vi "test.vi"() -> ()   [LabVIEW 2017]
uses:
  <vilib>/myRIO/Common/Instrument Driver Framework/myRIO v1.0/Encoder/typedefs/Encoder Signal Mode.ctl
  <vilib>/myRIO/Instrument Drivers/Onboard IO/PWM/typedefs/PWM Reference.ctl
  <vilib>/myRIO/Common/Instrument Driver Framework/Utilities/typedefs/myRIO Generic Hardware Reference.ctl
  <vilib>/myRIO/Common/Instrument Driver Framework/Utilities/typedefs/Hardware Version Enum.ctl
  <vilib>/myRIO/Common/Instrument Driver Framework/Utilities/typedefs/myRIO v1.0 Reference.ctl
  <vilib>/myRIO/Common/Instrument Driver Framework/Utilities/typedefs/Generic FPGA Reference.ctl
  <vilib>/myRIO/Common/Instrument Driver Framework/myRIO v1.0/PWM/typedefs/PWM Channels Enum.ctl
  <vilib>/myRIO/Instrument Drivers/Onboard IO/PWM/typedefs/PWM Configuration.ctl
  <vilib>/userdefined/High Color/nirio_resource_hc.ctl
  <vilib>/myRIO/Instrument Drivers/Onboard IO/DIO/typedefs/DIO Reference.ctl
  <vilib>/myRIO/Common/Instrument Driver Framework/myRIO v1.0/DIO/typedefs/DIO Channels List.ctl
  <vilib>/myRIO/Common/Instrument Driver Framework/myRIO v1.0/DIO/typedefs/DIO Channels Enum.ctl
  <vilib>/myRIO/Common/Instrument Driver Framework/Utilities/vis/Is FPGA Ref Available.vi
  <vilib>/myRIO/Common/Instrument Driver Framework/myRIO v1.0/PWM/vis/myRIO v1.1 Open PWM.vi
  <vilib>/myRIO/Instrument Drivers/Onboard IO/PWM/vis/Set Duty Cycle and Frequency.vi
  <vilib>/myRIO/Common/Instrument Driver Framework/myRIO v1.0/DIO/vis/myRIO v1.1 Open DIO.vi
  <vilib>/myRIO/Instrument Drivers/Onboard IO/DIO/vis/Write.vi
  <vilib>/myRIO/Common/Instrument Driver Framework/Utilities/vis/Validate Channels.vi
  <vilib>/myRIO/Common/Instrument Driver Framework/myRIO v1.0/PWM/vis/myRIO v1.0 Reserve PWM.vi
  <vilib>/myRIO/Common/Instrument Driver Framework/myRIO v1.0/DIO/vis/myRIO v1.0 Reserve DIO.vi
  <vilib>/myRIO/Common/Instrument Driver Framework/myRIO v1.0/Encoder/vis/myRIO v1.0 Close Encoder.vi
  <vilib>/myRIO/Common/Instrument Driver Framework/myRIO v1.0/UART/vis/myRIO v1.0 Close UART.vi
  <vilib>/myRIO/Common/Instrument Driver Framework/myRIO v1.0/PWM/vis/myRIO v1.0 Build MUX Configuration PWM.vi
  <vilib>/myRIO/Common/Instrument Driver Framework/myRIO v1.0/Resource Manager/vis/myRIO v1.0 Reserve Channel List.vi
  <vilib>/myRIO/Common/Instrument Driver Framework/myRIO v1.0/DIO/vis/myRIO v1.0 Build MUX Configuration DIO.vi
  <vilib>/myRIO/Common/Instrument Driver Framework/myRIO v1.0/Encoder/vis/myRIO v1.0 Unreserve Encoder.vi
  <vilib>/myRIO/Common/Instrument Driver Framework/myRIO v1.0/Resource Manager/vis/myRIO v1.0 Create Configuration List.vi
  <vilib>/myRIO/Common/Instrument Driver Framework/myRIO v1.0/Resource Manager/vis/myRIO v1.0 Reserve Channel.vi
  <vilib>/myRIO/Common/Instrument Driver Framework/myRIO v1.0/Resource Manager/vis/myRIO v1.0 Unreserve Channel.vi
  <vilib>/myRIO/Common/Instrument Driver Framework/myRIO v1.0/Encoder/vis/myRIO v1.0 Build MUX Configuration Encoder.vi
  <vilib>/myRIO/Common/Instrument Driver Framework/myRIO v1.0/Resource Manager/vis/myRIO v1.0 Unreserve Channel List.vi
  <vilib>/myRIO/Common/Instrument Driver Framework/myRIO v1.0/Resource Manager/vis/myRIO v1.0 Build Mutex Name.vi
  <vilib>/Utility/error.llb/Error Cluster From Error Code.vi
  <vilib>/myRIO/Common/Instrument Driver Framework/myRIO v1.0/Encoder/vis/myRIO v1.0 Reset Encoder.vi
  <vilib>/Utility/VariantDataType/GetNumericInfo.vi
  <vilib>/myRIO/Common/Instrument Driver Framework/myRIO v1.0/myRIO v1.1 Open.vi
  <vilib>/myRIO/Common/Instrument Driver Framework/Utilities/vis/IO Manager.vi
  <vilib>/myRIO/Common/Instrument Driver Framework/Utilities/vis/Configuration Manager.vi
  <vilib>/myRIO/Common/Instrument Driver Framework/myRIO v1.0/Resource Manager/vis/myRIO v1.0 Configure IO.vi
  <vilib>/myRIO/Common/Instrument Driver Framework/myRIO v1.0/myRIO v1.0 Close.vi
  <vilib>/myRIO/Common/Instrument Driver Framework/myRIO v1.0/PWM/vis/myRIO v1.0 Write PWM.vi
  <vilib>/myRIO/Common/Instrument Driver Framework/myRIO v1.0/DIO/vis/myRIO v1.0 Write DIO.vi
  <vilib>/myRIO/Common/Instrument Driver Framework/myRIO v1.0/Encoder/vis/myRIO v1.0 Read Encoder.vi
  <vilib>/myRIO/Common/Instrument Driver Framework/myRIO v1.0/Encoder/vis/myRIO v1.0 Shutdown Encoder.vi
  <vilib>/myRIO/Common/Instrument Driver Framework/Utilities/vis/FPGA Ref Manager.vi
  <vilib>/myRIO/Common/Instrument Driver Framework/myRIO v1.0/myRIO v1.0 Reset FPGA.vi
  <vilib>/myRIO/Common/Instrument Driver Framework/myRIO v1.0/IRQ/vis/myRIO v1.0 IRQ Info FGV.vi
  <vilib>/myRIO/Common/Instrument Driver Framework/myRIO v1.0/IRQ/vis/myRIO v1.0 Timer IRQ Info FGV.vi
  <vilib>/myRIO/Common/Instrument Driver Framework/myRIO v1.0/IRQ/vis/myRIO v1.0 ISR Agent.vi
  <vilib>/myRIO/Express VI/Onboard IO/PWM/PWM Express VI.xnode
  <vilib>/myRIO/Instrument Drivers/Onboard IO/PWM/vis/myRIO PWM Open.xnode
  <vilib>/myRIO/Express VI/Onboard IO/DO/DO Express VI.xnode
  <vilib>/myRIO/Instrument Drivers/Onboard IO/DIO/vis/myRIO DIO Open.xnode
  <vilib>/myRIO/Instrument Drivers/Onboard IO/Encoder/Encoder.lvlib
  <vilib>/myRIO/Instrument Drivers/Utilities/Utilities.lvlib
  <vilib>/myRIO/Instrument Drivers/Onboard IO/DIO/DIO.lvlib
  <vilib>/myRIO/Instrument Drivers/Onboard IO/PWM/PWM.lvlib
panel:
  in  "directionG":bool=TRUE
  in  "directionM":bool=TRUE
  in  "iterations":i32=5
  in  "frames to pass":i32=100
  in  "offset":i32=50
  in  "def it":i32=100
  in  "iterations control":i32=10
  out "ArrG_enc_val":i32[](array[numeric])
  out "ArrM_enc_val":i32[](array[numeric])
  in  "stop":bool
  in  "G+":bool
  in  "G-":bool
  in  "M+":bool
  in  "M-":bool
  out "M_enc_value":i32
  in  "Reset M_enc":bool
  out "G_enc_value":i32
  in  "Reset G_enc":bool
  in  "M/G_PWM":dbl=0.5
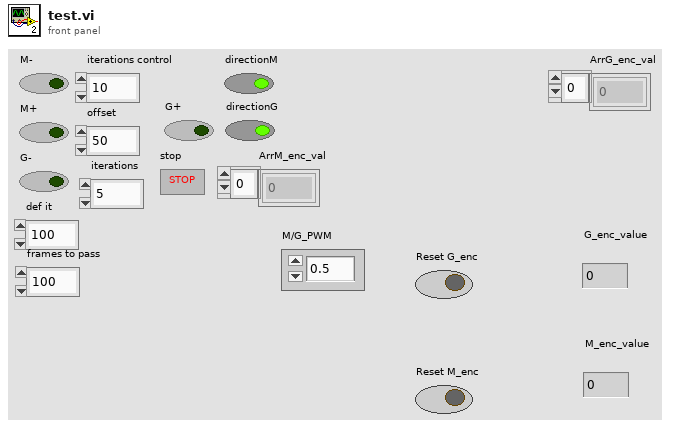
[diagram p1: front panel]
types:
  T1 = typedef "Encoder Signal Mode.ctl" = enum16{"Quadrature phase signal", "Step and direction signal"}
  T2 = typedef "Encoder.lvlib/Encoder Reference.ctl" = cluster{"myRIO Reference":T3, "Encoder Channels Enum":T7}
  T3 = typedef "myRIO Generic Hardware Reference.ctl" = cluster{"myRIO Model":T4, "myRIO Hardware Reference":T5}
  T4 = typedef "Hardware Version Enum.ctl" = enum16{"Unknown", "myRIO-1900", "myRIO-1950", "roboRIO", "NI ELVIS RIO CM"}
  T5 = typedef "myRIO v1.0 Reference.ctl" = cluster{"Generic FPGA Reference":T6, "Allow multiple opens":bool}
  T6 = typedef "Generic FPGA Reference.ctl" = refnum<k20>
  T7 = typedef "Encoder Channels Enum.ctl" = enum16{"Not Connected", "C/ENC0", "C/ENC1", "A/ENC", "B/ENC", "DIO/ENC0", "DIO/ENC1", "DIO/ENC2", "DIO/ENC3", "DIO/ENC4"}
  T8 = typedef "PWM.lvlib/PWM Reference.ctl" = cluster{"myRIO Reference":T3, "PWM Channels Enum":T9, "PWM Configuration":T10}
  T9 = typedef "PWM Channels Enum.ctl" = enum16{"Not Connected", "C/PWM0", "C/PWM1", "A/PWM0", "A/PWM1", "A/PWM2", "B/PWM0", "B/PWM1", "B/PWM2", "PWM/PWM0", "PWM/PWM1", "PWM/PWM2", "PWM/PWM3", "PWM/PWM4", "PWM/PWM5", "PWM/PWM6", "PWM/PWM7", "PWM/PWM8", "PWM/PWM9"}
  T10 = typedef "PWM.lvlib/PWM Configuration.ctl" = cluster{"Frequency":dbl, "Duty Cycle":dbl}
  T11 = typedef "nirio_resource_hc.ctl" = tag
  T12 = typedef "DIO.lvlib/DIO Reference.ctl" = cluster{"myRIO Reference":T3, "DIO Channels List":T13}
  T13 = typedef "DIO Channels List.ctl" = T14[]
  T14 = typedef "DIO Channels Enum.ctl" = enum16{"Not Connected", "C/DIO0", "C/DIO1", "C/DIO2", "C/DIO3", "C/DIO4", "C/DIO5", "C/DIO6", "C/DIO7", "A/DIO0", "A/DIO1", "A/DIO2", "A/DIO3", "A/DIO4", "A/DIO5", "A/DIO6", "A/DIO7", "A/DIO8", "A/DIO9", "A/DIO10", "A/DIO11", "A/DIO12", "A/DIO13", "A/DIO14", "A/DIO15", "B/DIO0", "B/DIO1", "B/DIO2", "B/DIO3", "B/DIO4", "B/DIO5", "B/DIO6", "B/DIO7", "B/DIO8", "B/DIO9", "B/DIO10", "B/DIO11", "B/DIO12", "B/DIO13", "B/DIO14", "B/DIO15", "LED0", "LED1", "LED2", "LED3", "Button0", "DIO/DIO0", "DIO/DIO1", "DIO/DIO2", "DIO/DIO3", "DIO/DIO4", "DIO/DIO5", "DIO/DIO6", "DIO/DIO7", "DIO/DIO8", "DIO/DIO9", "SPI/CS0", "SPI/CS1", "SPI/CS2", "SPI/CS3", "LED RADIO (Green)", "LED RADIO (Red)", "LED COMM (Green)", "LED COMM (Red)", "LED MODE (Green)", "LED MODE (Red)"}
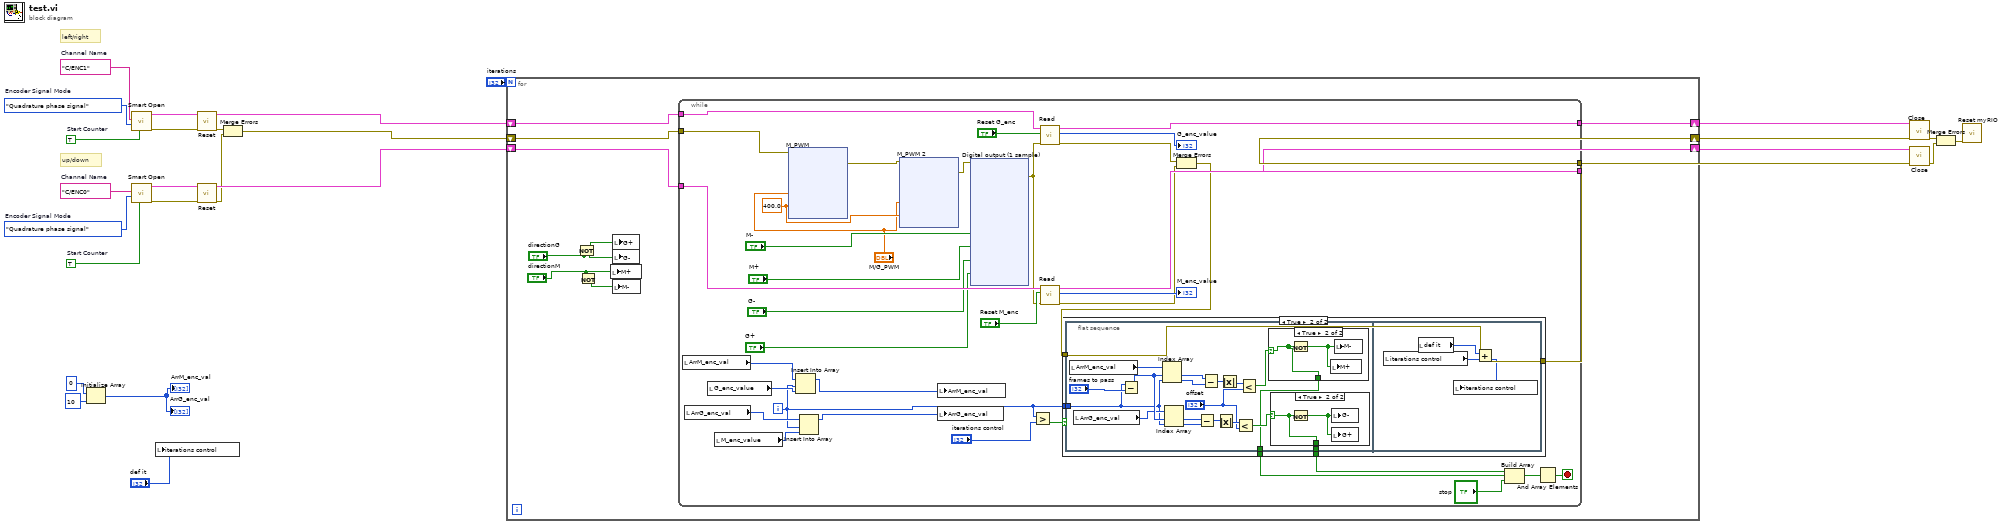
[diagram p0: block diagram]
diagram:
  w21 = TRUE  # Start Counter
  w25 = Encoder_Signal_Mode."Quadrature phase signal"  # Encoder Signal Mode
  w26 = tag "C/ENC1"  # Channel Name
  w22 = TRUE  # Start Counter
  w23 = Encoder_Signal_Mode."Quadrature phase signal"  # Encoder Signal Mode
  w24 = tag "C/ENC0"  # Channel Name
  # "left/right"
  # "up/down"
  n1 = Initialize Array(0 ("dimension size"), 10 ("dimension size")) -> (→"ArrM_enc_val" →"ArrG_enc_val":i32[])
  n2 = call <vilib>:"Smart Open.vi"("Start Counter"=w21, "Encoder Signal Mode"=w25, "Channel Name"=w26) -> ("error out"=w20:errorcluster, "Encoder Ref Out"=w19:T2)  [unwired: 7 in]
  n3 = call <vilib>:"Smart Open.vi"("Start Counter"=w22, "Encoder Signal Mode"=w23, "Channel Name"=w24) -> ("error out"=w17:errorcluster, "Encoder Ref Out"=w18:T2)  [unwired: 7 in]
  n4 = local write "iterations control"("def it") -> ()
  n5 = call <vilib>:"Reset.vi"("error in (no error)"=w20, "Encoder Ref In"=w19) -> ("error out"=w15:errorcluster, "Encoder Ref Out"=w14:T2)  [unwired: 8 in]
  n6 = call <vilib>:"Reset.vi"("error in (no error)"=w17, "Encoder Ref In"=w18) -> ("error out"=w12:errorcluster, "Encoder Ref Out"=w16:T2)  [unwired: 8 in]
  n7 = Merge Errors(w15, w12) -> (w13:errorcluster)
  n8 = for {
    N: "iterations" -> [_]
    shift-right: [w31] -> w9
    shift-left: w16 -> [w36]
    shift-right: [w33] -> w11
    shift-left: w14 -> [w35]
    shift-right: [w32] -> w10
    shift-left: w13 -> [w34]
    n9 = Not(x="directionG") -> (.not. x?=w28:bool)
    n10 = Not(x="directionM") -> (.not. x?=w27:bool)
    n11 = local write "M+"("directionM") -> ()
    n12 = local write "M-"(w27) -> ()
    n13 = local write "G+"(w28) -> ()
    n14 = local write "G-"("directionG") -> ()
    n15 = while {
      tunnel: w36 -> [w68]
      tunnel: w34 -> [w66]
      tunnel: w35 -> [w67]
      tunnel: [w65] -> w33
      tunnel: [w46] -> w32
      tunnel: [w64] -> w31
      i -> [w50]
      stop <- w41 stop-if-true
      w43 = 400.0 ("Frequency [Hz]")
      n16 = local read "ArrM_enc_val"() -> (w52:i32[])
      n17 = local read "ArrG_enc_val"() -> (w51:i32[])
      n18 = local read "G_enc_value"() -> (w55:i32)
      n19 = local read "M_enc_value"() -> (w56:i32)
      n20 = xnode "M_PWM"("Duty Cycle"="M/G_PWM", "Frequency [Hz]"=w43, "error in (no error)"=w66) -> ("error out"=w45:errorcluster)
      n21 = Insert Into Array(array=w52, index=w50, new element=w55) -> (w54:i32[])
      n22 = Insert Into Array(array=w51, index=w50, new element=w56) -> (w53:i32[])
      n23 = xnode "M_PWM 2"("Duty Cycle"="M/G_PWM", "Frequency [Hz]"=w43, "error in (no error)"=w45) -> ("error out"=w44:errorcluster)
      n24 = local write "ArrM_enc_val"(w54) -> ()
      n25 = local write "ArrG_enc_val"(w53) -> ()
      n26 = xnode "Digital output (1 sample)"("M+ (B/DIO5 (Pin 21))"="M-", "M- (B/DIO6 (Pin 23))"="M+", "G+ (B/DIO7 (Pin 25))"="G-", "G- (B/DIO13 (Pin 26))"="G+", "error in (no error)"=w44) -> ("error out"=w61:errorcluster)
      n27 = Greater?(x=w50, y="iterations control") -> (0:w48:bool)
      n28 = call <vilib>:"Read.vi"("error in (no error)"=w61, "Reset Counter"="Reset G_enc", "Encoder Ref In"=w67) -> ("error out"=w62:errorcluster, "Counter Value"=→"G_enc_value":i32, "Encoder Ref Out"=w65:T2)  [unwired: 4 in, 2 out]
      n29 = call <vilib>:"Read.vi"("error in (no error)"=w61, "Reset Counter"="Reset M_enc", "Encoder Ref In"=w68) -> ("error out"=w63:errorcluster, "Counter Value"=→"M_enc_value":i32, "Encoder Ref Out"=w64:T2)  [unwired: 4 in, 2 out]
      n30 = Merge Errors(w62, w63) -> (w47:errorcluster)
      n31 = case shown="True" w48 {
        selector: w48 -> [w108 _]
        tunnel: w50 -> [_ w113]
        tunnel: w47 -> [w109 w112]
        tunnel: [w109 w112] -> w46
        tunnel: [w108 w111] -> w39
        tunnel: [w108 w110] -> w38
        frame False {
        }
        frame True {
          n32 = flat-sequence {
            tunnel: w113 -> [w127]
            tunnel: [w115] -> w111
            tunnel: [w114] -> w110
            frame #0 {
              n33 = local read "ArrM_enc_val"() -> (w131:i32[])
              n34 = local read "ArrG_enc_val"() -> (w128:i32[])
              n35 = Subtract(x=w127, y="frames to pass") -> (x-y=w129:i32)
              n36 = Index Array(array=w131, index #1=w129, index #2=w127) -> (element #1=w126:i32, element #2=w125:i32)
              n37 = Index Array(array=w128, index #1=w129, index #2=w127) -> (element #1=w119:i32, element #2=w120:i32)
              n38 = Subtract(x=w119, y=w120) -> (x-y=w122:i32)
              n39 = Subtract(x=w126, y=w125) -> (x-y=w124:i32)
              n40 = Absolute Value(x=w122) -> (abs(x)=w121:i32)
              n41 = Absolute Value(x=w124) -> (abs(x)=w123:i32)
              n42 = Less?(x=w121, y="offset") -> (x < y?=w116:bool)
              n43 = Less?(x=w123, y="offset") -> (x < y?=w117:bool)
              n44 = case shown="True" w117 {
                selector: w117 -> [w135 w136]
                tunnel: [w135 w136] -> w115
                frame False {
                }
                frame True {
                  n45 = Not(x=w136) -> (.not. x?=w137:bool)
                  n46 = local write "M+"(w137) -> ()
                  n47 = local write "M-"(w137) -> ()
                }
              }
              n48 = case shown="True" w116 {
                selector: w116 -> [w132 w133]
                tunnel: [w132 w133] -> w114
                frame False {
                }
                frame True {
                  n49 = Not(x=w133) -> (.not. x?=w134:bool)
                  n50 = local write "G-"(w134) -> ()
                  n51 = local write "G+"(w134) -> ()
                }
              }
            }
            frame #1 {
              n52 = local read "iterations control"() -> (w140:i32)
              n53 = local read "def it"() -> (w138:i32)
              n54 = Add(x=w138, y=w140) -> (x+y=w139:i32)
              n55 = local write "iterations control"(w139) -> ()
            }
          }
        }
      }
      n56 = Build Array(w38, w39, "stop") -> (w37:bool[])
      n57 = And Array Elements(Boolean array=w37) -> (logical AND=w41:bool)
    }
  }
  n58 = call <vilib>:"Close.vi"("error in (no error)"=w10, "Encoder Ref In"=w11) -> ("error out"=w8:errorcluster)  [unwired: 9 in]
  n59 = call <vilib>:"Close.vi"("error in (no error)"=w10, "Encoder Ref In"=w9) -> ("error out"=w6:errorcluster)  [unwired: 9 in]
  n60 = Merge Errors(w8, w6) -> (w7:errorcluster)
  n61 = call <vilib>:"Reset myRIO.vi"("error in (no error)"=w7) -> ()  [unwired: 10 in, 1 out]
